vi "Clone Base.vi"(6 "Max Bits":i32=-1, 8 "error in (no error)":errorcluster, 10 "From":refnum<class "Packet.lvclass">, 11 "Packet in":refnum<class "Packet.lvclass">) -> (0 "error out":errorcluster, 3 "Packet out":refnum<class "Packet.lvclass">)   [LabVIEW 2020, in "Packet.lvclass"]
uses:
  Packet.lvclass
  Packet.lvclass/Packet.ctl
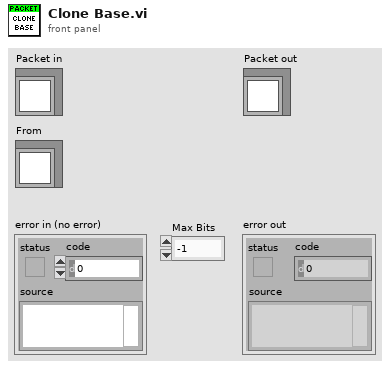
[diagram p1: front panel]
types:
  T1 = typedef "Type.ctl" = enum8{"Unknown", "NA 1", "NA 2", "NA 3", "Literal", "NA 5", "NA 6"}
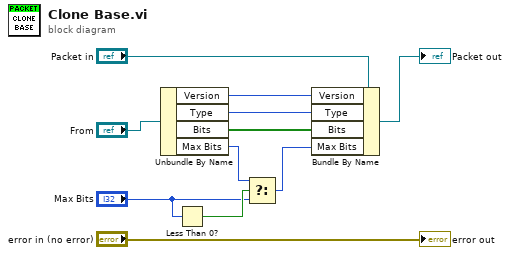
[diagram p0: block diagram]
diagram:
  n1 = Unbundle By Name("From") -> ("Version"=w7:u8, "Type"=w6:T1, "Bits"=w5:bool[], "Max Bits"=w4:i32)
  n2 = Less Than 0?(x="Max Bits") -> (x < 0?=w3:bool)
  n3 = Select(t=w4, s=w3, f="Max Bits") -> (s? t:f=w1:i32)
  n4 = Bundle By Name(cluster="Packet in", "Version"=w7, "Type"=w6, "Bits"=w5, "Max Bits"=w1) -> (→"Packet out":refnum<class "Packet.lvclass">)
  "error out" <- "error in (no error)"
